vi "Interface_Asset_Map Status.vi"(8 "error in (no error)":errorcluster, 11 "EnergyStorage_Virtual in":refnum<class "EnergyStorage_Virtual.lvclass">) -> (0 "error out":errorcluster, 3 "EnergyStorage_Virtual out":refnum<class "EnergyStorage_Virtual.lvclass">)   [LabVIEW 2015, in "EnergyStorage_Virtual.lvclass"]
uses:
  EnergyStorage_Virtual.lvclass
  EnergyStorage_Status.ctl
  EnergyStorage.lvclass
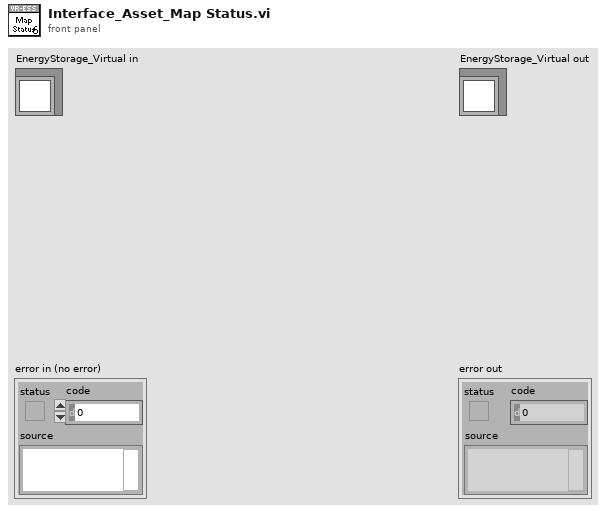
[diagram p1: front panel]
types:
  T1 = typedef "EnergyStorage.lvclass/EnergyStorage_Status.ctl" = cluster{"kW":dbl, "SOC":dbl}
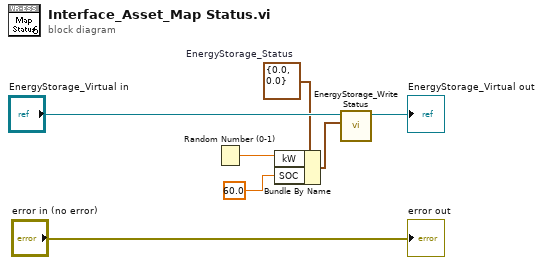
[diagram p0: block diagram]
diagram:
  w4 = T1 {"kW"=0.0, "SOC"=0.0}  # EnergyStorage_Status
  n1 = Random Number (0-1)() -> (number: 0 to 1=w2:dbl)
  n2 = Bundle By Name(cluster=w4, "kW"=w2, "SOC"=60.0) -> (w5:T1)
  n3 = call-dynamic "EnergyStorage_Write Status.vi"("EnergyStorage_Status"=w5, "EnergyStorage in"="EnergyStorage_Virtual in") -> ("EnergyStorage out"=→"EnergyStorage_Virtual out":refnum<class "EnergyStorage_Virtual.lvclass">)  [unwired: 9 in]
  "error out" <- "error in (no error)"
